vi "PidHmiReadInputRegistr.vi"(11 "register values":u16[](array[numeric])) -> (2 "number":sgl, 3 "Numeric":sgl)   [LabVIEW 2018, in "Pid.lvlib"]
uses:
  Pid.lvlib
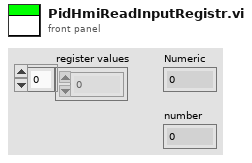
[diagram p1: front panel]
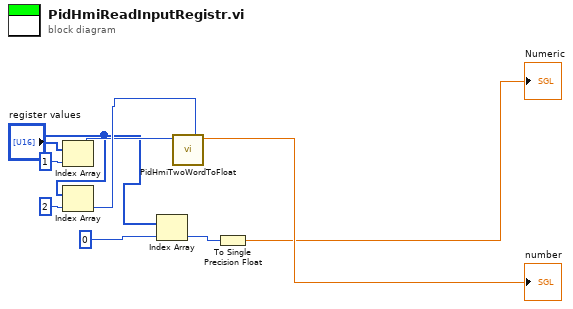
[diagram p0: block diagram]
diagram:
  n1 = Index Array(array="register values", index=1) -> (element=w8:u16)
  n2 = Index Array(array="register values", index=2) -> (element=w9:u16)
  n3 = Index Array(array="register values", index=0) -> (element=w6:u16)
  n4 = call "PidHmiTwoWordToFloat.vi"("register 2"=w9, "register 1"=w8) -> ("number"=→"number":sgl)  [unwired: 9 in]
  n5 = To Single Precision Float(number=w6) -> (single precision float=→"Numeric":sgl)
